vi "Acquire.vi"(8 "error in (no error)":errorcluster, 9 "Data Queue":T1, 10 "Data Notifier":T2, 11 "Hardware Resources in":T3={"Data source"=enum."Serial port", "Connection info"={"VISA resource name"="COM 1", "Baud rate"=9600, "data bits"=8, "stop bits"=0, "parity (0:none)"=enum."None", "flow control (0:none)"=0, "timeout (10sec)"=10000, "termination char\n(0xA = '\\n' = LF) "=10, "Enable Termination\nChar (T)"=TRUE}, "Protocol info"={"Temination char"=255, "Escape char"=254}, "Internet server"={"Web page telemetry"="", "Web page gps"=""}, "Data format"=enum."IDRA data"} {"Connection info"."flow control (0:none)" items=["None", "XON/XOFF", "RTS/CTS", "XON/XOFF & RTS/CTS", "DTR/DSR", "XON/XOFF & DTR/DSR"]}) -> (0 "error out":errorcluster, 3 "Hardware Resources out":T3={"Data source"=enum."Serial port", "Connection info"={"VISA resource name"="COM 1", "Baud rate"=9600, "data bits"=8, "stop bits"=0, "parity (0:none)"=enum."None", "flow control (0:none)"=0, "timeout (10sec)"=10000, "termination char\n(0xA = '\\n' = LF) "=10, "Enable Termination\nChar (T)"=TRUE}, "Protocol info"={"Temination char"=255, "Escape char"=254}, "Internet server"={"Web page telemetry"="", "Web page gps"=""}, "Data format"=enum."IDRA data"} {"Connection info"."flow control (0:none)" items=["None", "XON/XOFF", "RTS/CTS", "XON/XOFF & RTS/CTS", "DTR/DSR", "XON/XOFF & DTR/DSR"]})   [LabVIEW 2015, in "Acquisition.lvlib"]
doc: "Perform the acquisition. Replace the contents of this diagram with calls to acquisition hardware."
uses:
  Acquisition.lvlib
  Hardware Configuration.ctl
  controls/Data notifier.ctl
  Generic data packet.ctl
  My Graphs/Gps Map Graph coordinates.ctl
  controls/Data queue.ctl
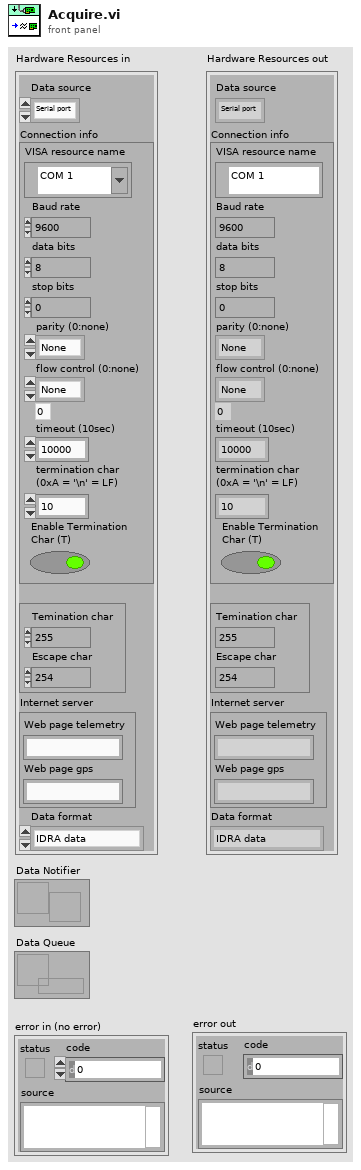
[diagram p1: front panel]
types:
  T1 = typedef "Data queue.ctl" = refnum<queue>
  T2 = typedef "Data notifier.ctl" = refnum<notifier>
  T3 = typedef "Acquisition.lvlib/Hardware Configuration.ctl" = cluster{"Data source":enum16{"Serial port", "Simulated data", "Web page JSON"}, "Connection info":cluster{"VISA resource name":refnum<visa-resource-name>, "Baud rate":u32, "data bits":u16, "stop bits":u16, "parity (0:none)":enum16{"None", "Odd", "Even", "Mark", "Space"}, "flow control (0:none)":u16, "timeout (10sec)":u32, "termination char\n(0xA = '\\n' = LF) ":u8, "Enable Termination\nChar (T)":bool}, "Protocol info":cluster{"Temination char":u8, "Escape char":u8}, "Internet server":cluster{"Web page telemetry":string, "Web page gps":string}, "Data format":enum16{"IDRA data", "XAM data"}}
  T4 = typedef "Acquisition.lvlib/Generic data packet.ctl" = cluster{"Content type":enum16{"None", "Telemetria", "GPS"}, "GPS":T5, "Telemetria":cluster{"Data format":enum16{"IDRA data", "XAM data"}, "Data":variant}}
  T5 = typedef "Gps Map Graph coordinates.ctl" = cluster{"Latitude":dbl, "Longitude":dbl}
  T6 = enum16{"Serial port", "Simulated data", "Web page JSON"}
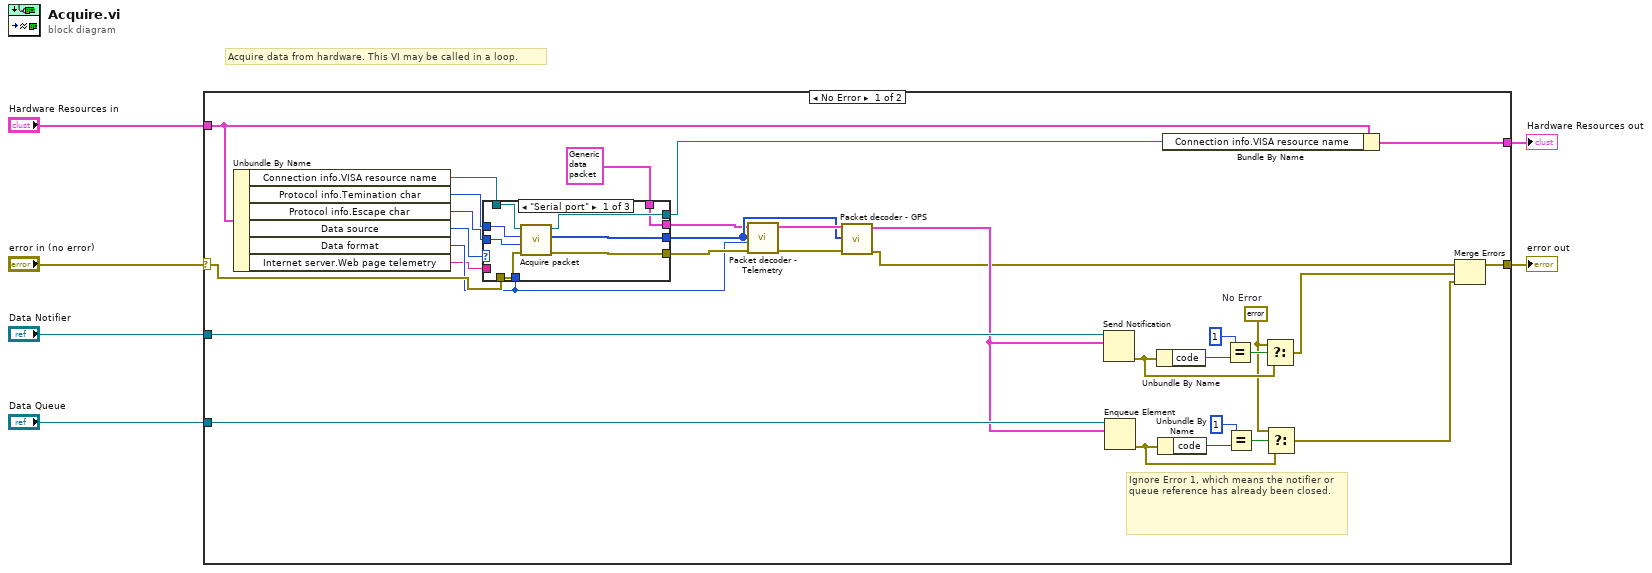
[diagram p0: block diagram]
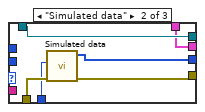
[diagram p2: hidden frame]
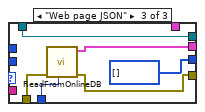
[diagram p3: hidden frame]
diagram:
  # "Acquire data from hardware. This VI may be called in a loop."
  n1 = case shown="No Error" "error in (no error)" {
    selector: "error in (no error)" -> [w29 w59]
    tunnel: [w37 w59] -> w5
    tunnel: "Hardware Resources in" -> [w36 w60]
    tunnel: [w38 w60] -> w3
    tunnel: "Data Notifier" -> [w35 _]
    tunnel: "Data Queue" -> [w32 _]
    frame No Error {
      w10 = errorcluster {"status"=FALSE, "code"=0, "source"=""}  # No Error
      # "Ignore Error 1, which means the notifier or queue reference has already been closed."
      n2 = Unbundle By Name(w36) -> ("Connection info.VISA resource name"=w31:refnum<visa-resource-name>, "Protocol info.Temination char"=w28:u8, "Protocol info.Escape char"=w27:u8, "Data source"=w20:T6, "Data format"=w19:enum16{"IDRA data", "XAM data"}, "Internet server.Web page telemetry"=w9:string)
      n3 = case shown="\"Serial port\"" w20 {
        tunnel: w31 -> [w46 w52 w58]
        tunnel: [w45 w52 w58] -> w30
        tunnel: w29 -> [w44 w51 w56]
        tunnel: w28 -> [w43 _ _]
        tunnel: w27 -> [w42 _ _]
        tunnel: [w41 w50 w57] -> w26
        tunnel: [w40 w49 u8[] [] ("Array")] -> w21
        tunnel: w19 -> [_ w48 w53]
        tunnel: w9 -> [_ _ _]
        tunnel: T4 {"Content type"=enum."None", "GPS"={"Latitude"=0.0, "Longitude"=0.0}, "Telemetria"={"Data format"=enum."IDRA data", "Data"=variant}} -> [w39 w47 _]
        tunnel: [w39 w47 w54] -> w7
        frame "Serial port" {
          n4 = call "Acquire packet.vi"("error in (no error)"=w44, "Escape"=w42, "Termination"=w43, "VISA resource name in"=w46) -> ("error out"=w41:errorcluster, "Packet"=w40:u8[], "VISA resource name out"=w45:refnum<visa-resource-name>)  [unwired: 5 in]
        }
        frame "Simulated data" {
          n5 = call "Simulated data.vi"("error in"=w51, "Data format"=w48) -> ("error out"=w50:errorcluster, "Array"=w49:u8[])  [unwired: 8 in]
        }
        frame "Web page JSON" {
          n6 = call "ReadFromOnlineDB.vi"("Data format"=w53, "error in"=w56) -> ("error out"=w57:errorcluster, "Output packet"=w54:T4)  [unwired: 8 in]
        }
      }
      n7 = call "Packet decoder - Telemetry.vi"("error in (no error)"=w26, "Data format"=w19, "Packet array"=w21, "Input packet"=w7) -> ("error out"=w23:errorcluster, "Output packet"=w25:T4)  [unwired: 5 in, 1 out]
      n8 = call "Packet decoder - GPS.vi"("error in (no error)"=w23, "Packet array"=w21, "Input packet"=w25) -> ("error out"=w22:errorcluster, "Output packet"=w24:T4)  [unwired: 6 in, 1 out]
      n9 = Send Notification(notification=w24, notifier=w35) -> (error out=w15:errorcluster)  [unwired: 1 in, 1 out]
      n10 = Enqueue Element(queue=w32, element=w24) -> (error out=w14:errorcluster)  [unwired: 2 in, 2 out]
      n11 = Unbundle By Name(w15) -> ("code"=w18:i32)
      n12 = Unbundle By Name(w14) -> ("code"=w11:i32)
      n13 = Bundle By Name(cluster=w36, "Connection info.VISA resource name"=w30) -> (w38:T3)
      n14 = Equal?(x=1, y=w18) -> (x = y?=w16:bool)
      n15 = Equal?(x=1, y=w11) -> (x = y?=w13:bool)
      n16 = Select(t=w10, s=w16, f=w15) -> (s? t:f=w34:errorcluster)
      n17 = Select(t=w10, s=w13, f=w14) -> (s? t:f=w33:errorcluster)
      n18 = Merge Errors(w22, w34, w33) -> (w37:errorcluster)
    }
    frame Error {
    }
  }
  "Hardware Resources out" <- w3
  "error out" <- w5
